vi "Initialize.vi"(8 "error in (no error)":errorcluster, 11 "Door Interlocks in":refnum<class "Door Interlocks.lvclass">) -> (0 "error out":errorcluster, 3 "Door Interlocks out":refnum<class "Door Interlocks.lvclass">)   [LabVIEW 2020, in "Door Interlocks.lvclass"]
uses:
  Door Interlocks.lvclass
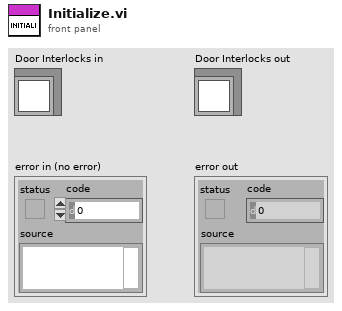
[diagram p1: front panel]
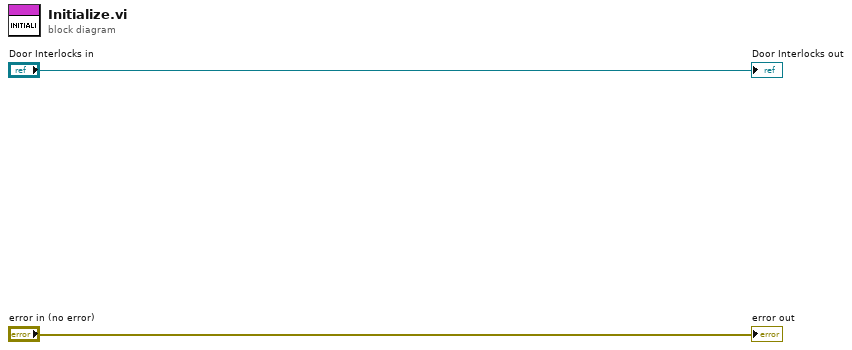
[diagram p0: block diagram]
diagram:
  "error out" <- "error in (no error)"
  "Door Interlocks out" <- "Door Interlocks in"
